vi "TestStand - Start Modal Dialog.vi"(0 "Sequence Context In":T1, 11 "error in (no error)":errorcluster) -> (4 "Sequence Context Out":T1, 6 "Modal ID":i32, 8 "VI Originally Open":bool, 10 "Should Abort":bool, 15 "error out":errorcluster)   [LabVIEW 2010]
doc: "Makes the calling dialog box VI modal to the TestStand main application window."
uses:
  6.0/DifferentStdPrototype/LabVIEW Test - Sequence Context.ctl
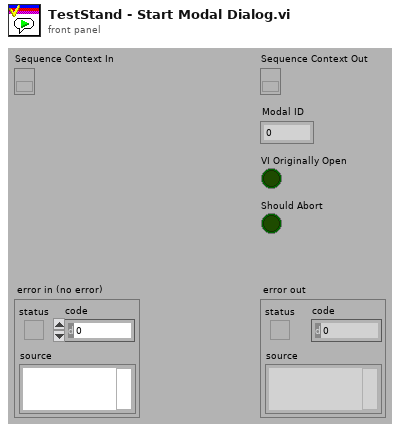
[diagram p1: front panel]
types:
  T1 = typedef "LabVIEW Test - Sequence Context.ctl" = refnum<k7>
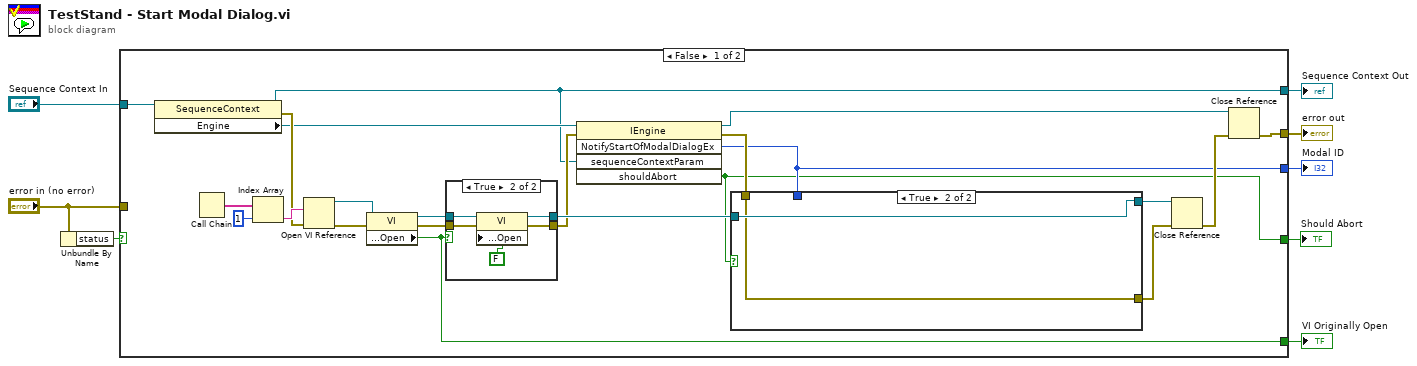
[diagram p0: block diagram]
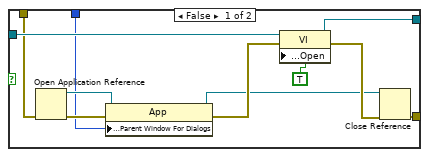
[diagram p2: hidden frame]
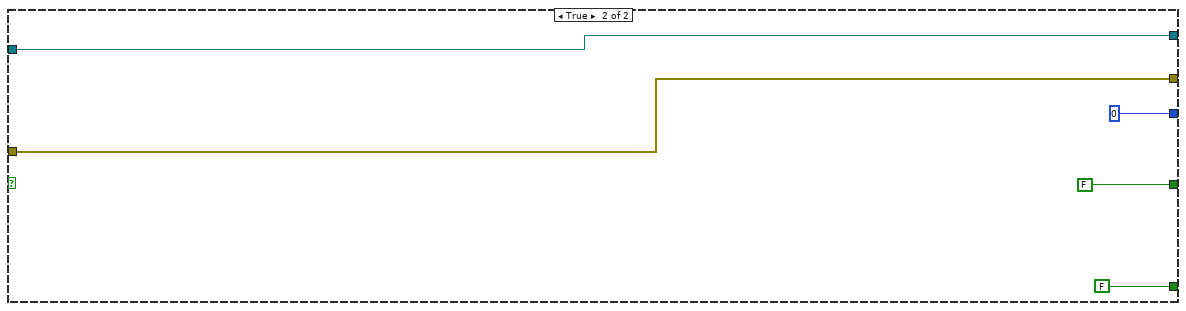
[diagram p4: hidden frame]
diagram:
  n1 = Unbundle By Name("error in (no error)") -> ("status"=w3:bool)
  n2 = case shown="False" w3 {
    tunnel: "Sequence Context In" -> [w23 w52]
    tunnel: [w15 w55] -> w7
    tunnel: [w11 0 ("NotifyStartOfModalDialog")] -> w6
    tunnel: [w14 FALSE ("Front Panel.Open")] -> w5
    tunnel: "error in (no error)" -> [_ w55]
    tunnel: [w10 w52] -> w2
    tunnel: [w9 FALSE ("Should Abort")] -> w1
    frame False {
      n3 = property class="SequenceContext"(reference=w23) -> (reference out=w10:T1, error out=w22:errorcluster, "Engine"=w12:refnum<k7>)  [unwired: 1 in]
      n4 = Call Chain() -> (call chain=w30:string[])
      n5 = Index Array(array=w30, index=1 ("Index")) -> (element=w28:string)
      n6 = Open VI Reference(vi path=w28, error in (no error)=w22) -> (vi reference=w26:refnum<vi>, error out=w27:errorcluster)  [unwired: 4 out]
      n7 = property class="VI"(reference=w26, error in=w27) -> (reference out=w24:refnum<vi>, error out=w25:errorcluster, "Front Panel Window:Open"=w14:bool)
      n8 = case shown="True" w14 {
        tunnel: [w45 w47] -> w13
        tunnel: w25 -> [w45 w50]
        tunnel: [w44 w48] -> w21
        tunnel: w24 -> [w44 w49]
        frame False {
        }
        frame True {
          n9 = property class="VI"(reference=w49, error in=w50, "Front Panel Window:Open"=FALSE) -> (reference out=w48:refnum<vi>, error out=w47:errorcluster)
        }
      }
      n10 = invoke class="IEngine" method="NotifyStartOfModalDialogEx"(reference=w12, error in=w13, "sequenceContextParam"=w10) -> (reference out=w16:refnum<k7>, error out=w20:errorcluster, "NotifyStartOfModalDialogEx"=w11:i32, "shouldAbort"=w9:bool)  [unwired: 2 in, 1 out]
      n11 = case shown="True" w9 {
        tunnel: w21 -> [w41 w43]
        tunnel: w20 -> [w40 w42]
        tunnel: [w35 w42] -> w19
        tunnel: [w34 w43] -> w18
        tunnel: w11 -> [w31 _]
        frame False {
          n12 = Open Application Reference(8:w40) -> (0:w39:errorcluster, 3:w38:refnum<vi>)  [unwired: 3 out]
          n13 = property class="App"(reference=w38, error in=w39, "Application:Parent Window For Dialogs"=w31) -> (reference out=w32:refnum<vi>, error out=w37:errorcluster)
          n14 = property class="VI"(reference=w41, error in=w37, "Front Panel Window:Open"=TRUE) -> (reference out=w34:refnum<vi>, error out=w33:errorcluster)
          n15 = Close Reference(reference=w32, error in (no error)=w33) -> (error out=w35:errorcluster)
        }
        frame True {
        }
      }
      n16 = Close Reference(reference=w18, error in (no error)=w19) -> (error out=w17:errorcluster)
      n17 = Close Reference(reference=w16, error in (no error)=w17) -> (error out=w15:errorcluster)
    }
    frame True {
    }
  }
  "error out" <- w7
  "Modal ID" <- w6
  "VI Originally Open" <- w5
  "Sequence Context Out" <- w2
  "Should Abort" <- w1
